vi "Set PU_CTRL.vi"(8 "error in (no error)":errorcluster, 10 "Configure NAU7802 CTRL0":T1, 11 "NAU7802 in":refnum<class "Adafruit NAU7802 24bit Strain Gauge.lvclass">) -> (0 "error out":errorcluster, 3 "NAU7802 out":refnum<class "Adafruit NAU7802 24bit Strain Gauge.lvclass">)   [LabVIEW 2020, in "CTI-Peripheral.lvlib" / "Adafruit NAU7802 24bit Strain Gauge.lvclass"]
uses:
  Adafruit NAU7802 24bit Strain Gauge.lvclass
  Private/ConfigDataCTRL0.ctl
  Adafruit NAU7802 24bit Strain Gauge.lvclass/Adafruit NAU7802 24bit Strain Gauge.ctl
  CTI/I2C Connection/I2C Connection.lvclass/I2C Connection.ctl
  CTI/Session/I2C Write Data.vi
  CTI/Session/I2C Read Data.vi
  CTI/I2C Connection/I2C Connection.lvclass
panel:
  out "Data":string
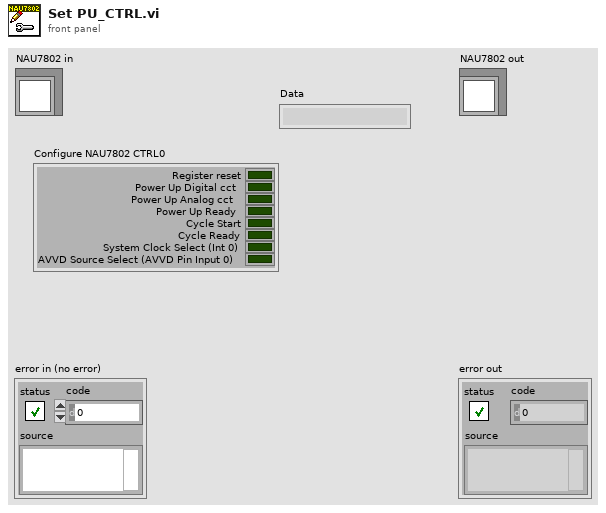
[diagram p1: front panel]
types:
  T1 = typedef "CTI-Peripheral.lvlib/Adafruit NAU7802 24bit Strain Gauge.lvclass/ConfigDataCTRL0.ctl" = cluster{"Register reset":bool, "Power Up Digital cct":bool, "Power Up Analog cct":bool, "Power Up Ready":bool, "Cycle Start":bool, "Cycle Ready":bool, "System Clock Select (Int 0)":bool, "AVVD Source Select (AVVD Pin Input 0)":bool}
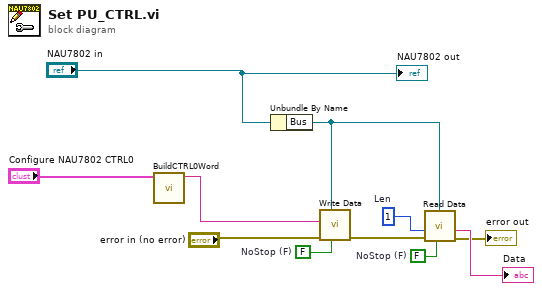
[diagram p0: block diagram]
diagram:
  w8 = FALSE  # NoStop (F)
  w9 = u8 1  # Len
  w10 = FALSE  # NoStop (F)
  n1 = call "BuildCTRL0Word.vi"("Configure NAU7802 CTRL0"="Configure NAU7802 CTRL0") -> ("string"=w2:string)  [unwired: 10 in]
  n2 = Unbundle By Name("NAU7802 in") -> ("Bus"=w4:refnum<class "I2C Connection.lvclass">)
  n3 = call "Write Data.vi"("NoStop (F)"=w10, "I2C Connection"=w4, "error in (no error)"="error in (no error)", "Data"=w2) -> ("error out"=w7:errorcluster)  [unwired: 7 in]
  n4 = call "Read Data.vi"("NoStop (F)"=w8, "I2C Connection"=w4, "error in (no error)"=w7, "Len"=w9) -> ("error out"=→"error out":errorcluster, "Data"=→"Data":string)  [unwired: 6 in]
  "NAU7802 out" <- "NAU7802 in"
